vi "ma_Check Block Size (2ch).vi"(6 "caller VI name":string, 7 "averaging parameters":T1={"averaging mode"=enum."No averaging", "weighting mode"=enum."Exponential", "number of averages"=10} {"number of averages" min=1}, 8 "error in":errorcluster, 9 "restart averaging (F)":bool, 10 "time signal Y":waveform(dbl), 11 "time signal X":waveform(dbl)) -> (0 "error out":errorcluster, 3 "force restart averaging":bool)   [LabVIEW 2020, in "NI_MAPro.lvlib"]
uses:
  NI_MAPro.lvlib
  NI_MABase.lvlib
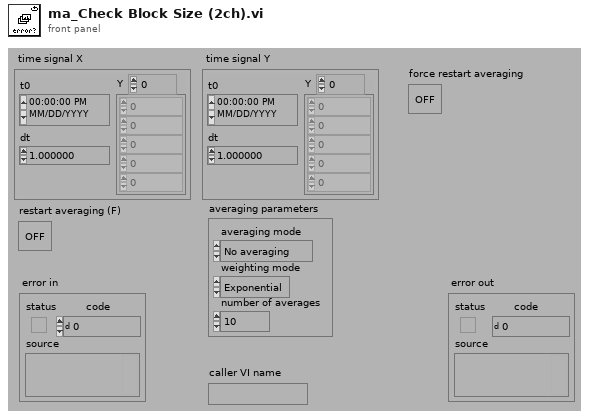
[diagram p1: front panel]
types:
  T1 = cluster{"averaging mode":enum16{"No averaging", "Vector averaging", "RMS averaging", "Peak hold"}, "weighting mode":enum16{"Linear", "Exponential"}, "number of averages":u32}
  T2 = enum16{"No averaging", "Vector averaging", "RMS averaging", "Peak hold"}
  T3 = cluster{"status":bool, "code":i32, "caller VI name":string}
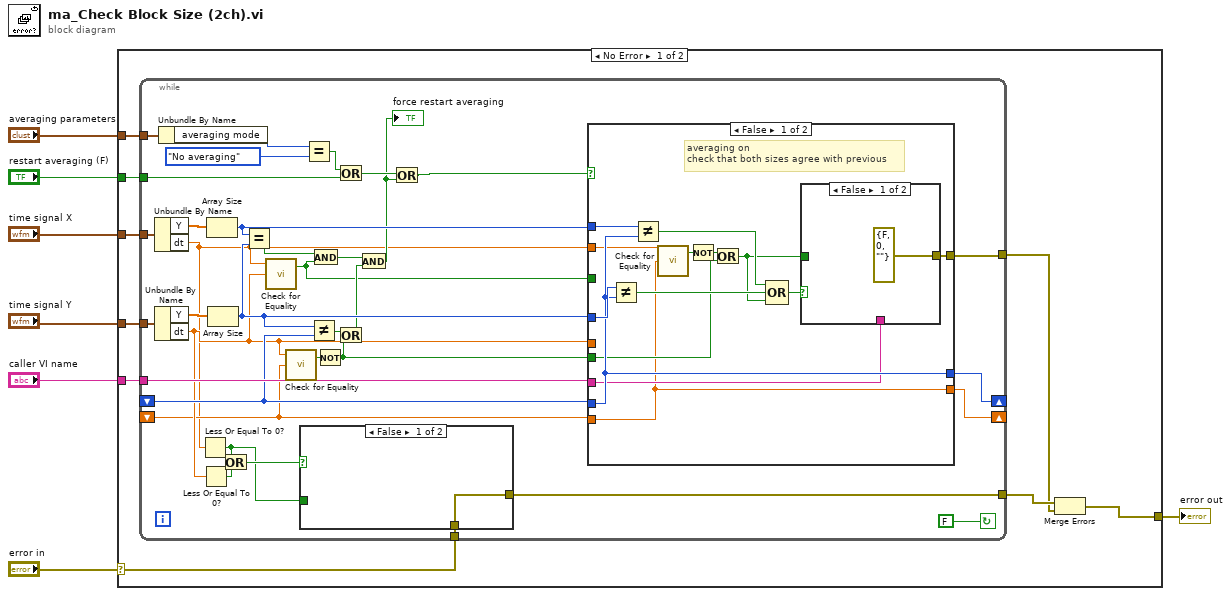
[diagram p0: block diagram]
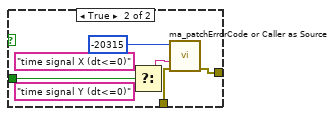
[diagram p2: hidden frame]
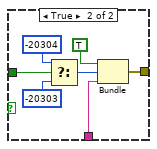
[diagram p3: hidden frame]
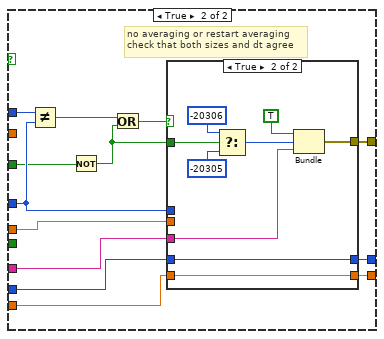
[diagram p4: hidden frame]
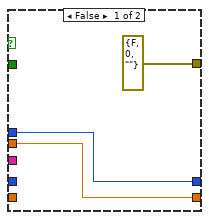
[diagram p5: hidden frame]
diagram:
  n1 = case shown="No Error" "error in" {
    selector: "error in" -> [w8 w107]
    tunnel: [w9 w107] -> w7
    tunnel: "time signal Y" -> [w16 _]
    tunnel: "time signal X" -> [w15 _]
    tunnel: "restart averaging (F)" -> [w14 _]
    tunnel: "averaging parameters" -> [w13 _]
    tunnel: "caller VI name" -> [w12 _]
    frame No Error {
      n2 = while {
        tunnel: w12 -> [w39]
        tunnel: w13 -> [w42]
        tunnel: w14 -> [w43]
        tunnel: w15 -> [w44]
        tunnel: w16 -> [w45]
        tunnel: [w38] -> w10
        shift-left: _ -> [w21]
        shift-right: [w40] -> _
        shift-left: _ -> [w34]
        shift-right: [w41] -> _
        tunnel: [w25] -> w11
        tunnel: w8 -> [w17]
        stop <- FALSE continue-if-true
        n3 = Unbundle By Name(w44) -> ("Y"=w50:dbl[], "dt"=w18:dbl)
        n4 = Unbundle By Name(w45) -> ("Y"=w49:dbl[], "dt"=w22:dbl)
        n5 = Unbundle By Name(w42) -> ("averaging mode"=w47:T2)
        n6 = Less Or Equal To 0?(x=w18) -> (x <= 0?=w24:bool)
        n7 = Less Or Equal To 0?(x=w22) -> (x <= 0?=w26:bool)
        n8 = Array Size(array=w50) -> (size(s)=w37:i32)
        n9 = Array Size(array=w49) -> (size(s)=w35:i32)
        n10 = Or(x=w24, y=w26) -> (x .or. y?=w27:bool)
        n11 = Equal?(x=w37, y=w35) -> (x = y?=w36:bool)
        n12 = call "Check for Equality.vi"("n2"=w22, "n1"=w18) -> ("equal?"=w20:bool)  [unwired: 1 in, 1 out]
        n13 = call "Check for Equality.vi"("n2"=w21, "n1"=w22) -> ("equal?"=w23:bool)  [unwired: 1 in, 1 out]
        n14 = case shown="False" w27 {
          tunnel: [w52 w54] -> w25
          tunnel: w24 -> [_ w57]
          tunnel: w17 -> [w52 w53]
          frame False {
          }
          frame True {
            n15 = Select(t="time signal X (dt<=0)", s=w57, f="time signal Y (dt<=0)") -> (s? t:f=w55:string)
            n16 = call "ma_patchErrorCode or Caller as Source.vi"("error in (no error)"=w53, "string to append to source"=w55, "error code"=-20315 ("code")) -> ("error out"=w54:errorcluster)  [unwired: 1 in, 7 out]
          }
        }
        n17 = Equal?(x=w47, y=T2."No averaging" ("averaging mode")) -> (x = y?=w46:bool)
        n18 = Not Equal?(x=w35, y=w34) -> (x != y?=w33:bool)
        n19 = And(x=w36, y=w20) -> (x .and. y?=w32:bool)
        n20 = Not(x=w23) -> (.not. x?=w19:bool)
        n21 = Or(x=w46, y=w43) -> (x .or. y?=w29:bool)
        n22 = Or(x=w33, y=w19) -> (x .or. y?=w31:bool)
        n23 = And(x=w32, y=w31) -> (x .and. y?=w28:bool)
        "force restart averaging" <- w28
        n24 = Or(x=w29, y=w28) -> (x .or. y?=w30:bool)
        n25 = case shown="False" w30 {
          tunnel: w37 -> [w73 w94]
          tunnel: w18 -> [w63 _]
          tunnel: w35 -> [w72 w91]
          tunnel: w22 -> [_ w89]
          tunnel: w34 -> [w70 w88]
          tunnel: w21 -> [w62 w87]
          tunnel: [w70 w92] -> w41
          tunnel: [w62 w90] -> w40
          tunnel: w39 -> [w65 w85]
          tunnel: [w68 w84] -> w38
          tunnel: w20 -> [_ w83]
          tunnel: w19 -> [w64 _]
          frame False {
            # "averaging on\ncheck that both sizes agree with previous"
            n26 = Not Equal?(x=w72, y=w70) -> (x != y?=w69:bool)
            n27 = Not Equal?(x=w73, y=w70) -> (x != y?=w71:bool)
            n28 = call "Check for Equality.vi"("n2"=w62, "n1"=w63) -> ("equal?"=w60:bool)  [unwired: 1 in, 1 out]
            n29 = Not(x=w60) -> (.not. x?=w61:bool)
            n30 = Or(x=w61, y=w64) -> (x .or. y?=w67:bool)
            n31 = Compound Arithmetic op=OR(w71, w69, w67) -> (w66:bool)
            n32 = case shown="False" w66 {
              tunnel: [errorcluster {"status"=FALSE, "code"=0, "source"=""} ("error in") w77] -> w68
              tunnel: w67 -> [_ w76]
              tunnel: w65 -> [_ w75]
              frame False {
              }
              frame True {
                n33 = Select(t=-20304 ("code"), s=w76, f=-20303 ("code")) -> (s? t:f=w79:i32)
                n34 = Bundle("status"=TRUE, "code"=w79, "caller VI name"=w75) -> (w77:T3)  [unwired: 1 out]
              }
            }
          }
          frame True {
            # "no averaging or restart averaging\ncheck that both sizes and dt agree"
            n35 = Not Equal?(x=w94, y=w91) -> (x != y?=w93:bool)
            n36 = Not(x=w83) -> (.not. x?=w82:bool)
            n37 = Or(x=w93, y=w82) -> (x .or. y?=w86:bool)
            n38 = case shown="True" w86 {
              tunnel: [w97 w106] -> w92
              tunnel: w91 -> [w97 _]
              tunnel: [w96 w105] -> w90
              tunnel: w89 -> [w96 _]
              tunnel: w88 -> [_ w106]
              tunnel: w87 -> [_ w105]
              tunnel: w82 -> [_ w104]
              tunnel: [errorcluster {"status"=FALSE, "code"=0, "source"=""} ("error in") w99] -> w84
              tunnel: w85 -> [_ w98]
              frame False {
              }
              frame True {
                n39 = Select(t=-20306 ("code"), s=w104, f=-20305 ("code")) -> (s? t:f=w100:i32)
                n40 = Bundle("status"=TRUE, "code"=w100, "caller VI name"=w98) -> (w99:T3)  [unwired: 1 out]
              }
            }
          }
        }
      }
      n41 = Merge Errors(w11, w10) -> (w9:errorcluster)
    }
    frame Error {
    }
  }
  "error out" <- w7
